vi "Open.vi"(7 "Path":path, 8 "error in (no error)":errorcluster, 10 "Operation":T1, 11 "Data.TDMS in":refnum<class "Data.PG.lvclass">) -> (0 "error out":errorcluster, 3 "Data.TDMS out":refnum<class "Data.PG.lvclass">)   [LabVIEW 2020, in "Data.PG.lvclass"]
uses:
  Data.PG.lvclass
  C:/user/patrick/git/LV-to-ITX/src/Data/Data.lvclass
  Data/Typedefs/Operation--enum.ctl
  Data.PG.lvclass/Data.PG.ctl
  Data/Data.lvclass
  <vilib>/JDP Science/PostgreSQL Library/Connection/PQ Connection.lvclass
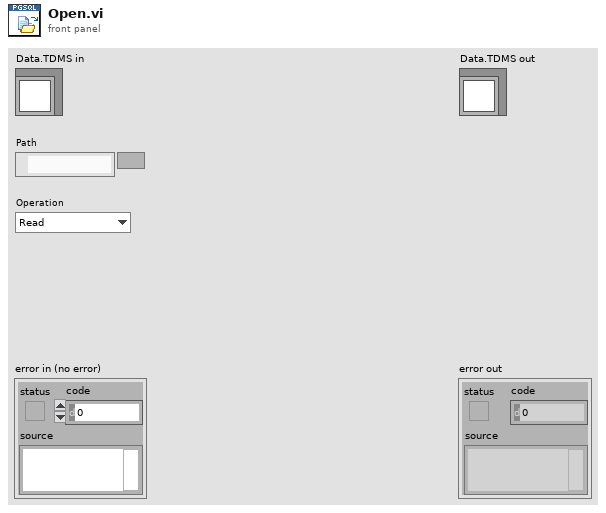
[diagram p1: front panel]
types:
  T1 = typedef "Data.lvclass/Operation--enum.ctl" = enum16{"Read", "Write", "Write + Append"}
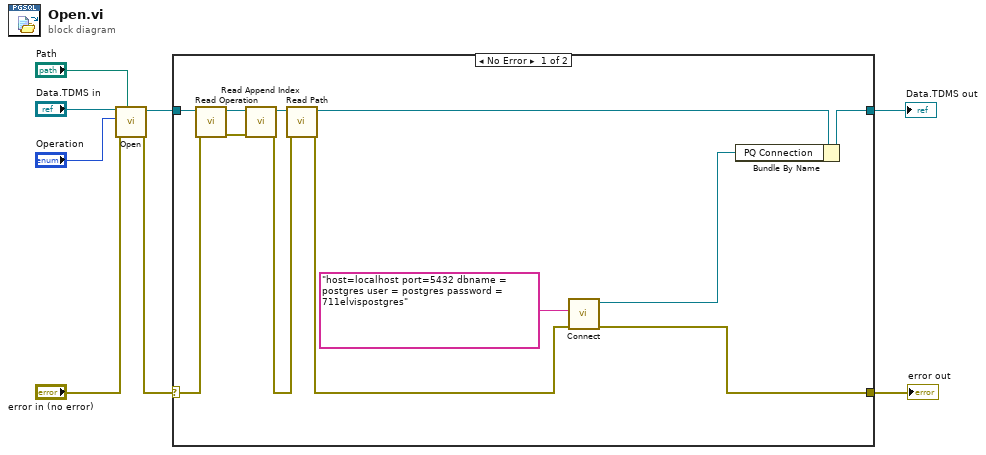
[diagram p0: block diagram]
diagram:
  n1 = call-parent "Open.vi"("Path"="Path", "error in (no error)"="error in (no error)", "Operation"="Operation", "Data in"="Data.TDMS in") -> ("error out"=w6:errorcluster, "Data out"=w4:refnum<class "Data.PG.lvclass">)  [unwired: 6 in]
  n2 = case shown="No Error" w6 {
    selector: w6 -> [w14 w22]
    tunnel: [w9 w22] -> w5
    tunnel: w4 -> [w16 w21]
    tunnel: [w19 w21] -> w3
    frame No Error {
      n3 = call "Read Operation.vi"("error in (no error)"=w14, "Data in"=w16) -> ("error out"=w13:errorcluster, "Data out"=w15:refnum<class "Data.PG.lvclass">)  [unwired: 7 in, 1 out]
      n4 = call "Read Append Index.vi"("error in (no error)"=w13, "Data in"=w15) -> ("error out"=w17:errorcluster, "Data out"=w18:refnum<class "Data.PG.lvclass">)  [unwired: 7 in, 1 out]
      n5 = call "Read Path.vi"("error in (no error)"=w17, "Data Save"=w18) -> ("error out"=w11:errorcluster, "Data Save out"=w20:refnum<class "Data.PG.lvclass">)  [unwired: 7 in, 1 out]
      n6 = call <vilib>:"Connect.vi"("error in (no error)"=w11, "Connection Strings"="host=localhost port=5432 dbname = postgres user = postgres password = 711elvispostgres" ("Connection Strings to access PostgreSQL")) -> ("error out"=w9:errorcluster, "PQ Connection out"=w10:refnum<class "PQ Connection.lvclass">)  [unwired: 8 in]
      n7 = Bundle By Name(cluster=w20, "PQ Connection"=w10) -> (w19:refnum<class "Data.PG.lvclass">)
    }
    frame Error {
    }
  }
  "error out" <- w5
  "Data.TDMS out" <- w3
